vi "Mpemba_HotColdWarm.vi"(6 "RN":sgl, 8 "X0":sgl=0.5, 11 "Ring":i16(ring) items=["Cold", "Warm", "Hot"]) -> (3 "Xpot":sgl)   [LabVIEW 2019]
uses:
  <vilib>/Platform/TimedLoop/XDataNode/timing_clust.ctl
  <vilib>/Platform/TimedLoop/XDataNode/nitl_modes.ctl
  <vilib>/Platform/TimedLoop/XDataNode/wakeup.ctl
  <vilib>/rvi/Emulation/niFpgaGetClockAttributes.vi
  <vilib>/rvi/Emulation/niFpgaSctlEmulationGetInTimedLoop.vi
  <vilib>/rvi/Emulation/niFpgaEmulationReportErrorSimple.vi
  <vilib>/rvi/Emulation/niFpgaCriticalErrorInLSC.vi
  <vilib>/Platform/TimedLoop/XDataNode/XDataNode.xnode
  <vilib>/Platform/TimedLoop/XDataNode/XDNodeRunTimeDep.lvlib
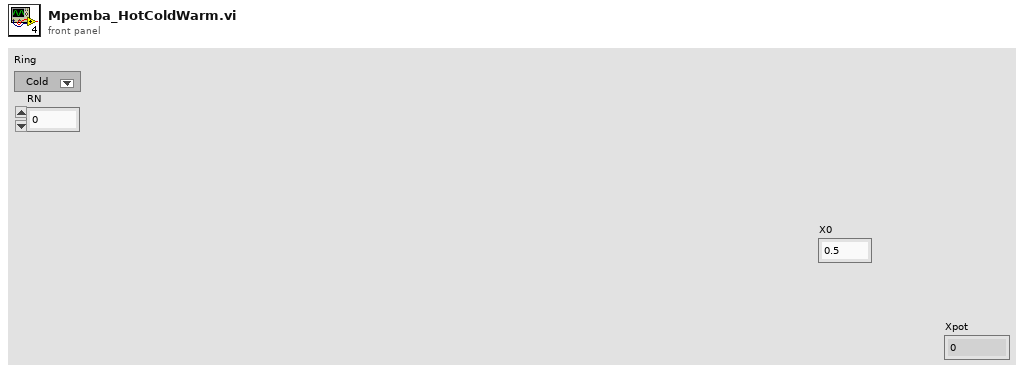
[diagram p1: front panel]
types:
  T1 = typedef "XDNodeRunTimeDep.lvlib/timing_clust.ctl" = cluster{"Expected End [f-1]":u64, "Actual End [f-1]":u64, "Finished Late? [f-1]":bool, "Expected End [i-1]":u64, "Actual End [i-1]":u64, "Finished Late? [i-1]":bool, "Expected Start [i]":u64, "Actual Start [i]":u64, "Expected Start [f]":u64, "Actual Start [f]":u64, "Source Name":string, "Structure Name":string, "Period":i64, "Deadline":i64, "Offset":i64, "Start":i64, "Priority":i32, "Timeout":i32, "Mode":T2, "Wakeup Reason":T3, "Error":errorcluster, "Source Type":string, "Secondary Source Type":string, "Global End Time":u64, "Global Start Time":u64, "Frame Duration":u64, "Iteration Duration":u64, "Assigned CPU":i32, "I/O Scan Engine Mode":u32}
  T2 = typedef "XDNodeRunTimeDep.lvlib/nitl_modes.ctl" = enum32{"No Change", "Process missed periods, maintain original phase", "Discard missed periods, maintain original phase", "Process missed periods, ignore original phase", "Discard missed periods, ignore original phase"}
  T3 = typedef "XDNodeRunTimeDep.lvlib/wakeup.ctl" = enum32{"Normal", "Aborted", "Asynchronous wakeup", "Timing source error", "Timed loop error", "Timeout"}
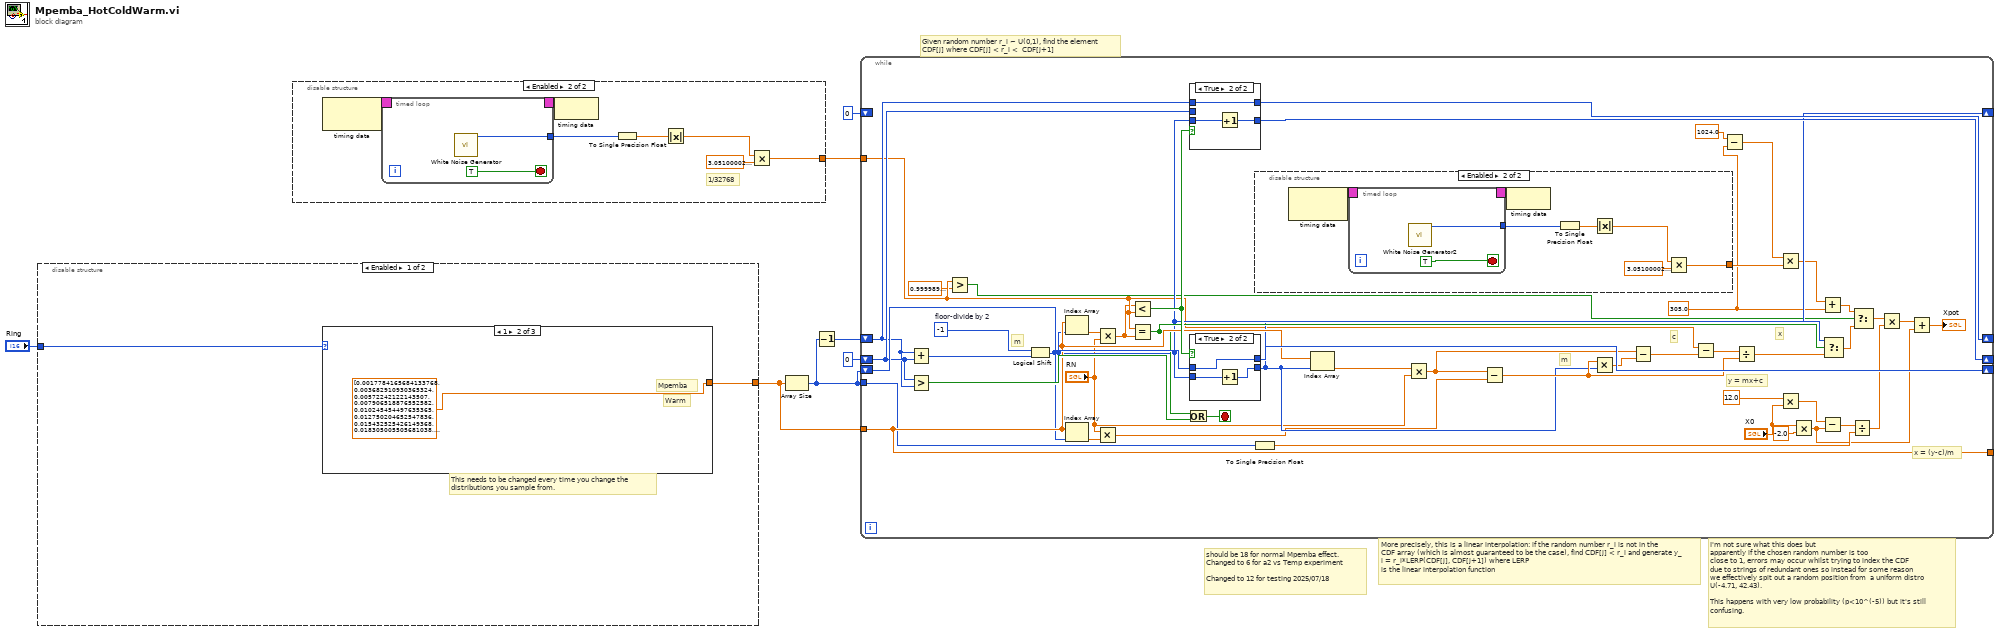
[diagram p0: block diagram]
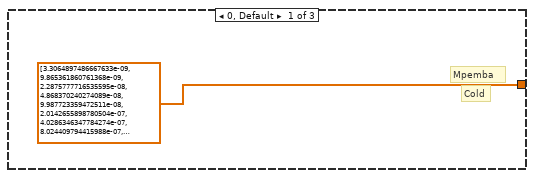
[diagram p2: hidden frame]
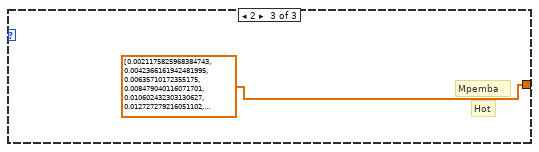
[diagram p3: hidden frame]
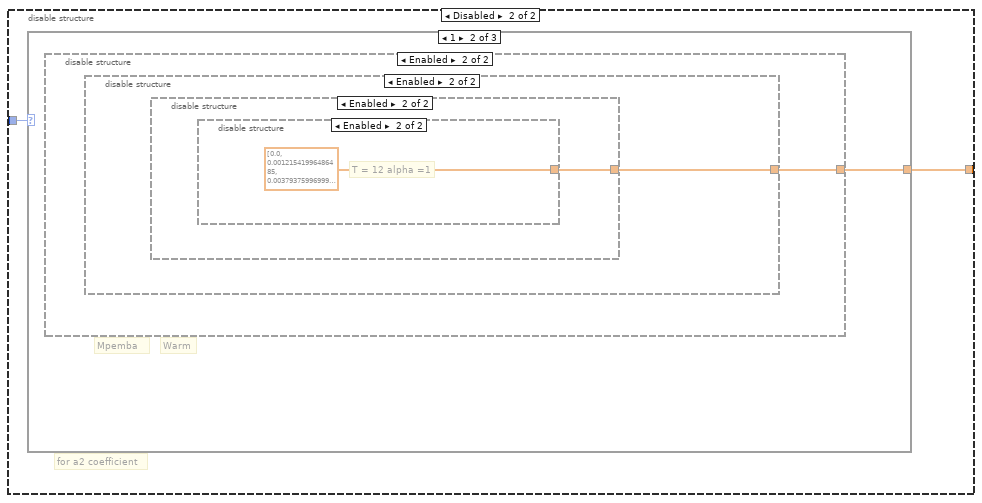
[diagram p4: hidden frame]
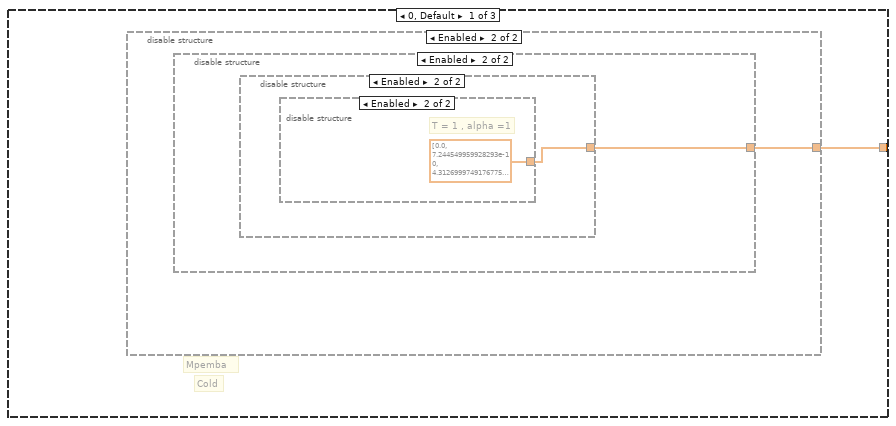
[diagram p5: hidden frame]
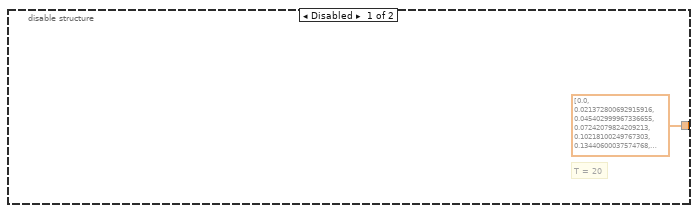
[diagram p6: hidden frame]
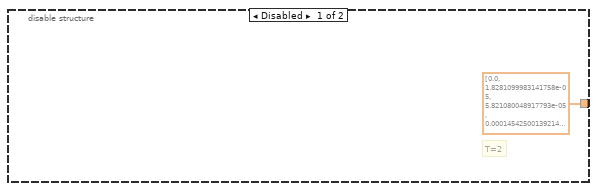
[diagram p7: hidden frame]
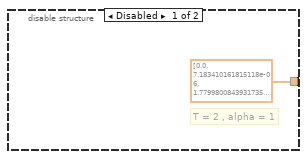
[diagram p8: hidden frame]
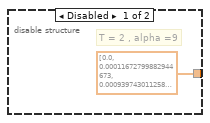
[diagram p9: hidden frame]
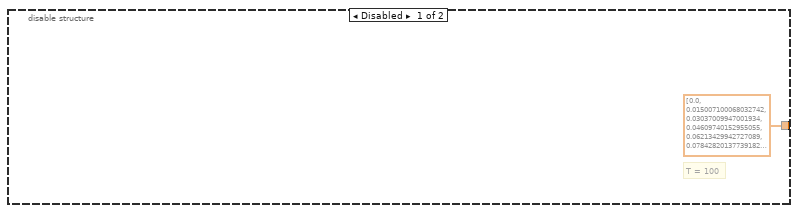
[diagram p10: hidden frame]
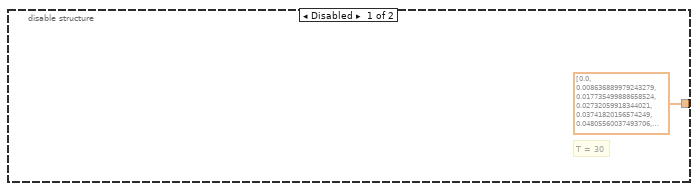
[diagram p11: hidden frame]
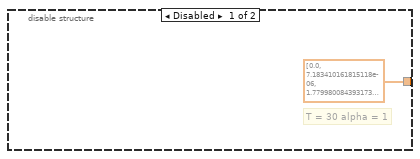
[diagram p12: hidden frame]
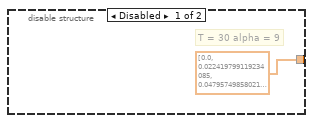
[diagram p13: hidden frame]
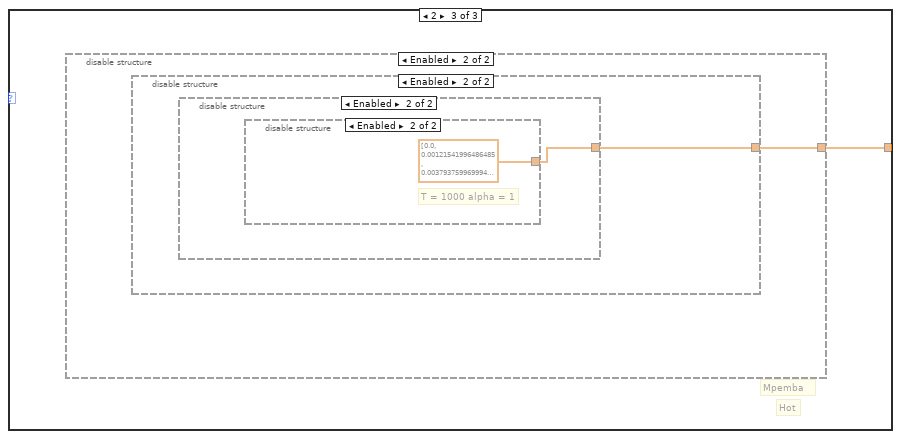
[diagram p14: hidden frame]
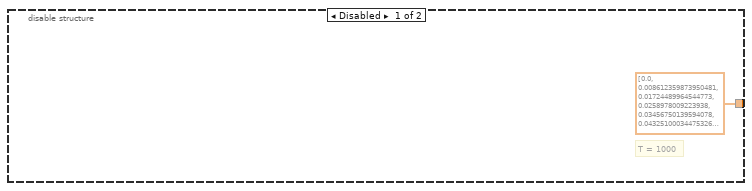
[diagram p15: hidden frame]
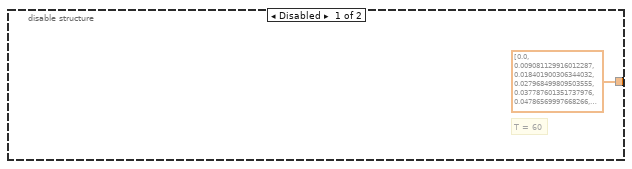
[diagram p16: hidden frame]
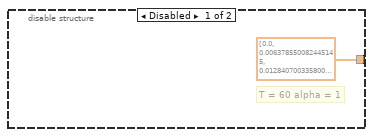
[diagram p17: hidden frame]
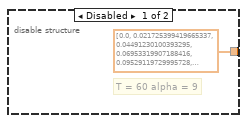
[diagram p18: hidden frame]
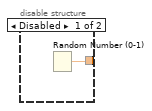
[diagram p19: hidden frame]
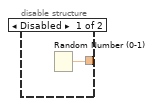
[diagram p20: hidden frame]
diagram:
  # "Given random number r_i ~ U(0,1), find the element\nCDF[j] where CDF[j] < r_i <  CDF[j+1]"
  # "I'm not sure what this does but\napparently if the chosen random number is too \nclose to 1, errors may occur whilst trying to index the CDF\ndue to strings of redundant ones so instead for some reason\nwe effectively spit out a random position from  a uniform distro\nU(-4.71, 42.43).\n\nThis happens with very low probability (p<10^(-5)) but it's still\nconfusing."
  # "More precisely, this is a linear interpolation: if the random number r_i is not in the\nCDF array (which is almost guaranteed to be the case), find CDF[j] < r_i and generate y_i = r_i*LERP(CDF[j], CDF[j+1]) where LERP\nis the linear interpolation function"
  # "should be 18 for normal Mpemba effect.\nChanged to 6 for a2 vs Temp experiment\n\nChanged to 12 for testing 2025/07/18"
  n1 = disable-structure shown="Enabled" {
    disable-tunnel: "Ring" -> [w9 w13]
    disable-tunnel: [w8 w14] -> w1
    frame Enabled {
      # "This needs to be changed every time you change the \ndistributions you sample from."
      n2 = case shown="1" w9 {
        tunnel: [sgl[] [3.3064897e-09, 9.865362e-09, 2.2875778e-08, 4.8683702e-08, 9.9877234e-08, 2.0142656e-07, 4.0286346e-07, 8.02441e-07, 1.5950573e-06, 3.1673194e-06, 6.286115e-06, 1.247267e-05, 2.4715764e-05, 4.8135003e-05, 9.1060996e-05, 0.00016657586, 0.0002942775, 0.00050219335, 0.0008286077, 0.0013234806, 0.0020490861, 0.0030795163, 0.004498784, 0.006397423, 0.008867702, 0.011997792, 0.015865415, 0.020531645, 0.026035521, 0.03239009, 0.039580304, 0.047562927, 0.0562685, 0.06560501, 0.075462855, 0.085720666, 0.0962513, 0.106927626, 0.11762765, 0.12823877, 0.13866088, 0.14880845, 0.15861152, 0.16801578, 0.17698202, 0.18548483, 0.19351119, 0.20105864, 0.20813352, 0.2147492, 0.22092445, 0.22668195, 0.23204707, 0.23704672, 0.24170859, 0.24606037, 0.25012928, 0.25394168, 0.25752282, 0.2608967, 0.26408604, 0.2671121, 0.2699949, 0.27275333, 0.27540496, 0.2779665, 0.28045377, 0.28288183, 0.28526524, 0.28761804, 0.2899542, 0.2922874, 0.29463166, 0.2970011, 0.29941046, 0.3018751, 0.30441135, 0.30703667, 0.30977, 0.31263185, 0.31564495, 0.31883422, 0.32222733, 0.3258551, 0.32975185, 0.33395582, 0.33850968, 0.34346086, 0.34886217, 0.354772, 0.36125463, 0.36838052, 0.37622622, 0.3848741, 0.3944119, 0.40493152, 0.4165278, 0.42929626, 0.44333023, 0.4587175, 0.4755356, 0.49384695, 0.5136926, 0.535086, 0.558006, 0.5823905, 0.60813034, 0.63506484, 0.6629795, 0.69160587, 0.72062594, 0.7496793, 0.77837545, 0.8063088, 0.83307797, 0.85830593, 0.8816607, 0.9028746, 0.92175883, 0.93821377, 0.95223135, 0.9638909, 0.9733483, 0.9808191, 0.9865588, 0.9908417, 0.9939414, 0.99611413, 0.9975871, 0.99855137, 0.9991601, 0.99953, 0.9997462, 0.9998674, 0.99993247, 0.99996597, 0.99998283, 0.99999136, 0.99999565, 0.9999978, 0.99999887, 0.99999946, 0.9999997, 0.9999999, 0.99999994, 0.99999994, 1.0, 1.0, 1.0, 1.0, 1.0, 1.0, 1.0, 1.0, 1.0, 1.0, 1.0, 1.0, 1.0, 1.0, 1.0, 1.0, 1.0, 1.0, 1.0, 1.0, 1.0, 1.0, 1.0, 1.0, 1.0, 1.0, 1.0, 1.0, 1.0, 1.0, 1.0, 1.0, 1.0, 1.0, 1.0, 1.0, 1.0, 1.0, 1.0, 1.0, 1.0, 1.0, 1.0, 1.0, 1.0, 1.0, 1.0, 1.0, 1.0, 1.0, 1.0, 1.0, 1.0, 1.0, 1.0, 1.0, 1.0, 1.0, 1.0, 1.0, 1.0, 1.0, 1.0, 1.0, 1.0, 1.0, 1.0, 1.0, 1.0, 1.0, 1.0, 1.0, 1.0, 1.0, 1.0, 1.0, 1.0, 1.0, 1.0, 1.0, 1.0, 1.0, 1.0, 1.0, 1.0, 1.0, 1.0, 1.0, 1.0, 1.0, 1.0, 1.0, 1.0, 1.0, 1.0, 1.0, 1.0, 1.0, 1.0, 1.0, 1.0, 1.0, 1.0, 1.0, 1.0, 1.0, 1.0, 1.0, 1.0, 1.0, 1.0, 1.0, 1.0, 1.0, 1.0, 1.0, 1.0, 1.0, 1.0, 1.0, 1.0, 1.0, 1.0, 1.0, 1.0, 1.0, 1.0, 1.0, 1.0, 1.0, 1.0, 1.0, 1.0, 1.0, 1.0, 1.0, 1.0, 1.0, 1.0, 1.0, 1.0, 1.0, 1.0, 1.0, 1.0, 1.0, 1.0, 1.0, 1.0, 1.0, 1.0, 1.0, 1.0, 1.0, 1.0, 1.0, 1.0, 1.0, 1.0, 1.0, 1.0, 1.0, 1.0, 1.0, 1.0, 1.0, 1.0, 1.0, 1.0, 1.0, 1.0, 1.0, 1.0, 1.0, 1.0, 1.0, 1.0, 1.0, 1.0, 1.0, 1.0, 1.0, 1.0, 1.0, 1.0, 1.0, 1.0, 1.0, 1.0, 1.0, 1.0, 1.0, 1.0, 1.0, 1.0, 1.0, 1.0, 1.0, 1.0, 1.0, 1.0, 1.0, 1.0, 1.0, 1.0, 1.0, 1.0, 1.0, 1.0, 1.0, 1.0, 1.0, 1.0, 1.0, 1.0, 1.0, 1.0, 1.0, 1.0, 1.0, 1.0, 1.0, 1.0, 1.0, 1.0, 1.0, 1.0, 1.0, 1.0, 1.0, 1.0, 1.0, 1.0, 1.0, 1.0, 1.0, 1.0, 1.0, 1.0, 1.0, 1.0, 1.0, 1.0, 1.0, 1.0, 1.0, 1.0, 1.0, 1.0, 1.0, 1.0, 1.0, 1.0, 1.0, 1.0, 1.0, 1.0, 1.0, 1.0, 1.0, 1.0, 1.0, 1.0, 1.0, 1.0, 1.0, 1.0, 1.0, 1.0, 1.0, 1.0, 1.0, 1.0, 1.0, 1.0, 1.0, 1.0, 1.0, 1.0, 1.0, 1.0, 1.0, 1.0, 1.0, 1.0, 1.0, 1.0, 1.0, 1.0, 1.0, 1.0, 1.0, 1.0, 1.0, 1.0, 1.0, 1.0, 1.0, 1.0, 1.0, 1.0, 1.0, 1.0, 1.0, 1.0, 1.0, 1.0, 1.0, 1.0, 1.0, 1.0, 1.0, 1.0, 1.0, 1.0, 1.0, 1.0, 1.0, 1.0, 1.0, 1.0, 1.0, 1.0, 1.0, 1.0, 1.0, 1.0, 1.0, 1.0, 1.0, 1.0, 1.0, 1.0, 1.0, 1.0, 1.0, 1.0, 1.0, 1.0, 1.0, 1.0, 1.0, 1.0, 1.0, 1.0, 1.0, 1.0, 1.0, 1.0, 1.0, 1.0, 1.0, 1.0, 1.0, 1.0, 1.0, 1.0, 1.0, 1.0, 1.0, 1.0, 1.0, 1.0, 1.0, 1.0, 1.0, 0.0, 0.0] ("Array") sgl[] [0.0017784166, 0.003682911, 0.005722421, 0.007906519, 0.0102454545, 0.012750205, 0.015432525, 0.018305006, 0.021381123, 0.024675317, 0.02820305, 0.031980872, 0.03602557, 0.040341295, 0.044926606, 0.049778376, 0.054891855, 0.060260758, 0.065877356, 0.07173262, 0.07781631, 0.084117144, 0.090622984, 0.09732092, 0.10419748, 0.11123878, 0.11843064, 0.12575877, 0.1332089, 0.14076687, 0.1484188, 0.15615115, 0.16395082, 0.17180526, 0.17970249, 0.1876312, 0.19558074, 0.20354122, 0.21150346, 0.21945906, 0.22740036, 0.23532051, 0.24321334, 0.25107348, 0.2588962, 0.2666775, 0.27441406, 0.2821032, 0.28974277, 0.29733124, 0.3048676, 0.31235138, 0.3197825, 0.32716137, 0.33448884, 0.34176603, 0.34899446, 0.356176, 0.3633127, 0.37040702, 0.37746152, 0.38447905, 0.39146265, 0.39841548, 0.40534094, 0.4122425, 0.41912377, 0.4259885, 0.43284047, 0.43968362, 0.44652188, 0.4533593, 0.46019995, 0.46704793, 0.47390732, 0.48078233, 0.48767704, 0.4945956, 0.5015421, 0.5085206, 0.5155351, 0.52258956, 0.52968794, 0.5368339, 0.54403114, 0.55128324, 0.5585935, 0.56596524, 0.57340133, 0.58090466, 0.58847773, 0.5961228, 0.6038418, 0.6116363, 0.6195075, 0.6274562, 0.6354827, 0.64358693, 0.6517681, 0.66002494, 0.6683555, 0.6767572, 0.68522686, 0.6937603, 0.70235276, 0.7109986, 0.7196914, 0.72842366, 0.7371872, 0.7459729, 0.7547705, 0.7635692, 0.7723569, 0.7811211, 0.78984797, 0.7985233, 0.80713195, 0.81565815, 0.82408583, 0.83239824, 0.84057844, 0.8486093, 0.8564739, 0.8641552, 0.8716366, 0.8789022, 0.8859366, 0.8927255, 0.8992556, 0.9055147, 0.91149247, 0.9171798, 0.92256963, 0.9276564, 0.9324368, 0.9369095, 0.9410861, 0.9449862, 0.9486281, 0.952029, 0.95520467, 0.9581701, 0.9609393, 0.9635251, 0.96593976, 0.96819454, 0.9703001, 0.9722662, 0.9741022, 0.9758166, 0.9774176, 0.97891253, 0.98030853, 0.9816121, 0.9828294, 0.98396605, 0.98502755, 0.9860187, 0.98694426, 0.9878086, 0.98861563, 0.9893693, 0.990073, 0.9907302, 0.99134386, 0.9919169, 0.992452, 0.9929517, 0.9934183, 0.993854, 0.99426085, 0.99464077, 0.9949956, 0.9953269, 0.9956362, 0.9959251, 0.99619484, 0.9964468, 0.996682, 0.99690163, 0.99710673, 0.9972983, 0.9974771, 0.9976442, 0.9978001, 0.9979457, 0.99808174, 0.9982087, 0.9983273, 0.99843806, 0.9985415, 0.998638, 0.99872816, 0.9988124, 0.998891, 0.9989644, 0.999033, 0.999097, 0.9991568, 0.99921256, 0.9992647, 0.99931335, 0.99935883, 0.9994013, 0.9994409, 0.9994779, 0.9995125, 0.99954474, 0.9995749, 0.99960303, 0.9996293, 0.9996539, 0.99967676, 0.99969816, 0.9997181, 0.9997368, 0.99975425, 0.9997705, 0.9997857, 0.9997999, 0.99981314, 0.9998255, 0.99983704, 0.9998478, 0.9998579, 0.9998673, 0.9998761, 0.9998843, 0.99989194, 0.9998991, 0.99990577, 0.999912, 0.99991786, 0.9999233, 0.99992836, 0.9999331, 0.99993753, 0.99994165, 0.9999455, 0.99994916, 0.9999525, 0.99995565, 0.9999586, 0.9999613, 0.9999639, 0.99996626, 0.9999685, 0.9999706, 0.9999725, 0.99997437, 0.99997604, 0.99997765, 0.99997914, 0.9999805, 0.9999818, 0.999983, 0.99998415, 0.99998516, 0.9999862, 0.99998707, 0.99998796, 0.99998873, 0.99998945, 0.99999017, 0.9999908, 0.9999914, 0.999992, 0.99999255, 0.999993, 0.9999935, 0.9999939, 0.99999434, 0.9999947, 0.99999505, 0.99999535, 0.9999957, 0.99999595, 0.99999624, 0.9999965, 0.9999967, 0.99999696, 0.99999714, 0.9999973, 0.9999975, 0.9999977, 0.9999978, 0.999998, 0.9999981, 0.9999982, 0.99999833, 0.99999845, 0.99999857, 0.9999986, 0.99999875, 0.9999988, 0.9999989, 0.999999, 0.99999905, 0.9999991, 0.99999917, 0.9999992, 0.9999993, 0.99999934, 0.99999934, 0.9999994, 0.99999946, 0.99999946, 0.9999995, 0.9999995, 0.9999996, 0.9999996, 0.99999964, 0.99999964, 0.9999997, 0.9999997, 0.9999997, 0.99999976, 0.99999976, 0.99999976, 0.99999976, 0.9999998, 0.9999998, 0.9999998, 0.9999998, 0.9999998, 0.9999999, 0.9999999, 0.9999999, 0.9999999, 0.9999999, 0.9999999, 0.9999999, 0.99999994, 0.99999994, 0.99999994, 0.99999994, 0.99999994, 0.99999994, 0.99999994, 0.99999994, 0.99999994, 0.99999994, 0.99999994, 0.99999994, 0.99999994, 0.99999994, 0.99999994, 0.99999994, 1.0, 1.0, 1.0, 1.0, 1.0, 1.0, 1.0, 1.0, 1.0, 1.0, 1.0, 1.0, 1.0, 1.0, 1.0, 1.0, 1.0, 1.0, 1.0, 1.0, 1.0, 1.0, 1.0, 1.0, 1.0, 1.0, 1.0, 1.0, 1.0, 1.0, 1.0, 1.0, 1.0, 1.0, 1.0, 1.0, 1.0, 1.0, 1.0, 1.0, 1.0, 1.0, 1.0, 1.0, 1.0, 1.0, 1.0, 1.0, 1.0, 1.0, 1.0, 1.0, 1.0, 1.0, 1.0, 1.0, 1.0, 1.0, 1.0, 1.0, 1.0, 1.0, 1.0, 1.0, 1.0, 1.0, 1.0, 1.0, 1.0, 1.0, 1.0, 1.0, 1.0, 1.0, 1.0, 1.0, 1.0, 1.0, 1.0, 1.0, 1.0, 1.0, 1.0, 1.0, 1.0, 1.0, 1.0, 1.0, 1.0, 1.0, 1.0, 1.0, 1.0, 1.0, 1.0, 1.0, 1.0, 1.0, 1.0, 1.0, 1.0, 1.0, 1.0, 1.0, 1.0, 1.0, 1.0, 1.0, 1.0, 1.0, 1.0, 1.0, 1.0, 1.0, 1.0, 1.0, 1.0, 1.0, 1.0, 1.0, 1.0, 1.0, 1.0, 1.0, 1.0, 1.0, 1.0, 1.0, 1.0, 1.0, 1.0, 1.0, 1.0, 1.0, 1.0, 1.0, 1.0, 1.0, 1.0, 1.0, 1.0, 1.0, 1.0, 1.0, 1.0, 1.0, 1.0, 1.0, 1.0, 1.0, 1.0, 1.0, 1.0, 1.0, 1.0, 1.0, 1.0, 1.0, 1.0, 1.0, 1.0, 1.0, 1.0, 1.0, 0.0, 0.0] ("Array") sgl[] [0.0021175826, 0.004236616, 0.0063571017, 0.00847904, 0.010602432, 0.012727279, 0.014853583, 0.016981343, 0.01911056, 0.021241236, 0.023373373, 0.02550697, 0.027642025, 0.029778464, 0.031916197, 0.03405514, 0.036195207, 0.038336314, 0.040478393, 0.04262136, 0.044765145, 0.046909686, 0.049054913, 0.051200762, 0.053347178, 0.0554941, 0.05764148, 0.05978926, 0.061937395, 0.06408584, 0.06623455, 0.068383485, 0.070532605, 0.072681874, 0.07483126, 0.07698074, 0.07913027, 0.08127982, 0.08342939, 0.08557893, 0.08772844, 0.089877896, 0.09202727, 0.09417655, 0.09632574, 0.09847481, 0.10062376, 0.10277257, 0.104921244, 0.107069775, 0.10921816, 0.11136639, 0.11351447, 0.1156624, 0.11781018, 0.11995781, 0.1221053, 0.12425265, 0.12639986, 0.12854694, 0.1306939, 0.13284075, 0.1349875, 0.13713415, 0.13928072, 0.14142722, 0.14357364, 0.14572002, 0.14786637, 0.15001267, 0.15215896, 0.15430526, 0.15645157, 0.15859789, 0.16074425, 0.16289066, 0.16503714, 0.16718368, 0.16933031, 0.17147705, 0.17362389, 0.17577085, 0.17791794, 0.18006518, 0.18221258, 0.18436013, 0.18650787, 0.18865578, 0.19080387, 0.19295216, 0.19510065, 0.19724934, 0.19939823, 0.20154734, 0.20369665, 0.20584618, 0.20799592, 0.21014586, 0.21229601, 0.21444635, 0.21659689, 0.21874762, 0.22089851, 0.22304955, 0.22520076, 0.2273521, 0.22950354, 0.23165509, 0.23380673, 0.2359584, 0.23811011, 0.24026182, 0.2424135, 0.24456514, 0.24671668, 0.24886808, 0.25101933, 0.25317037, 0.25532115, 0.25747165, 0.25962177, 0.26177153, 0.2639208, 0.26606962, 0.26821783, 0.27036545, 0.27251235, 0.27465847, 0.2768038, 0.2789482, 0.2810916, 0.28323394, 0.28537515, 0.2875151, 0.28965372, 0.2917909, 0.29392666, 0.29606092, 0.29819375, 0.3003251, 0.302455, 0.30458343, 0.30671042, 0.30883595, 0.31096002, 0.31308264, 0.3152038, 0.3173235, 0.31944177, 0.32155856, 0.3236739, 0.32578784, 0.3279003, 0.3300113, 0.33212087, 0.334229, 0.3363357, 0.33844092, 0.34054473, 0.34264708, 0.344748, 0.34684747, 0.34894553, 0.35104212, 0.35313728, 0.35523102, 0.35732335, 0.3594142, 0.36150363, 0.36359164, 0.36567822, 0.36776337, 0.3698471, 0.37192938, 0.37401026, 0.3760897, 0.37816772, 0.3802443, 0.3823195, 0.38439324, 0.38646558, 0.3885365, 0.39060602, 0.3926741, 0.39474076, 0.396806, 0.39886984, 0.40093225, 0.40299326, 0.40505287, 0.40711105, 0.40916783, 0.4112232, 0.41327718, 0.41532972, 0.41738087, 0.41943064, 0.421479, 0.42352593, 0.42557147, 0.4276156, 0.42965835, 0.4316997, 0.43373963, 0.43577817, 0.43781534, 0.43985108, 0.44188544, 0.4439184, 0.44595, 0.4479802, 0.450009, 0.45203638, 0.4540624, 0.45608705, 0.45811027, 0.46013215, 0.46215263, 0.4641717, 0.4661894, 0.46820575, 0.4702207, 0.47223428, 0.47424647, 0.47625726, 0.47826672, 0.48027477, 0.48228145, 0.4842868, 0.48629072, 0.48829326, 0.49029446, 0.49229428, 0.49429274, 0.49628985, 0.49828556, 0.5002799, 0.5022729, 0.50426453, 0.5062548, 0.5082437, 0.5102312, 0.5122174, 0.5142022, 0.51618564, 0.51816773, 0.5201485, 0.52212787, 0.5241059, 0.5260826, 0.5280579, 0.53003186, 0.5320045, 0.5339757, 0.53594565, 0.5379142, 0.53988147, 0.54184735, 0.54381186, 0.54577506, 0.5477369, 0.54969734, 0.55165654, 0.5536143, 0.5555708, 0.55752593, 0.5594797, 0.5614322, 0.5633833, 0.56533307, 0.56728154, 0.56922865, 0.5711744, 0.57311887, 0.575062, 0.5770038, 0.5789442, 0.5808833, 0.58282113, 0.5847576, 0.58669275, 0.58862656, 0.59055907, 0.59249026, 0.5944201, 0.59634864, 0.59827584, 0.6002017, 0.6021263, 0.60404956, 0.60597146, 0.6078921, 0.6098114, 0.6117294, 0.6136461, 0.6155614, 0.6174755, 0.6193882, 0.6212997, 0.62320983, 0.6251186, 0.62702614, 0.62893236, 0.63083726, 0.63274086, 0.63464314, 0.6365441, 0.6384438, 0.6403422, 0.6422393, 0.64413506, 0.64602953, 0.64792275, 0.64981467, 0.65170527, 0.65359455, 0.6554826, 0.6573693, 0.6592547, 0.66113883, 0.6630217, 0.6649033, 0.6667835, 0.66866255, 0.6705402, 0.6724166, 0.67429173, 0.6761656, 0.6780382, 0.6799094, 0.68177944, 0.68364817, 0.6855156, 0.68738174, 0.6892466, 0.6911102, 0.69297254, 0.6948336, 0.69669336, 0.6985519, 0.7004091, 0.7022651, 0.70411974, 0.7059732, 0.7078253, 0.7096762, 0.7115258, 0.7133742, 0.7152213, 0.71706706, 0.71891165, 0.7207549, 0.72259694, 0.7244377, 0.72627723, 0.7281155, 0.72995245, 0.7317882, 0.73362267, 0.7354559, 0.7372879, 0.7391186, 0.740948, 0.7427762, 0.74460316, 0.74642885, 0.74825335, 0.75007653, 0.75189847, 0.75371915, 0.75553864, 0.7573568, 0.7591738, 0.76098955, 0.76280403, 0.76461726, 0.76642925, 0.76824003, 0.7700495, 0.7718578, 0.77366483, 0.7754707, 0.7772752, 0.77907854, 0.78088063, 0.7826815, 0.7844811, 0.7862795, 0.7880767, 0.78987265, 0.79166734, 0.7934608, 0.79525304, 0.79704404, 0.79883385, 0.8006224, 0.80240977, 0.8041959, 0.8059808, 0.8077645, 0.80954695, 0.8113282, 0.81310815, 0.814887, 0.8166645, 0.8184409, 0.82021606, 0.82198995, 0.8237627, 0.82553416, 0.8273045, 0.82907355, 0.8308414, 0.83260804, 0.83437353, 0.8361378, 0.83790076, 0.8396626, 0.8414232, 0.8431826, 0.84494084, 0.8466978, 0.8484536, 0.8502082, 0.8519616, 0.8537138, 0.85546476, 0.85721457, 0.8589632, 0.86071056, 0.8624568, 0.8642018, 0.8659456, 0.8676882, 0.86942965, 0.87116987, 0.8729089, 0.8746468, 0.8763834, 0.8781189, 0.8798532, 0.88158625, 0.8833182, 0.88504887, 0.8867784, 0.88850677, 0.89023393, 0.89195997, 0.89368474, 0.8954084, 0.8971308, 0.89885205, 0.9005722, 0.90229106, 0.9040088, 0.90572536, 0.9074407, 0.90915495, 0.910868, 0.91257983, 0.91429055, 0.91600007, 0.9177084, 0.9194156, 0.9211216, 0.9228264, 0.9245301, 0.9262326, 0.92793393, 0.9296341, 0.9313331, 0.93303096, 0.93472767, 0.9364232, 0.9381175, 0.93981075, 0.94150275, 0.9431937, 0.9448834, 0.94657195, 0.94825935, 0.9499456, 0.9516307, 0.95331466, 0.9549975, 0.9566791, 0.9583596, 0.96003896, 0.9617171, 0.96339417, 0.96507007, 0.96674484, 0.9684184, 0.97009087, 0.9717622, 0.97343236, 0.97510135, 0.97676927, 0.978436, 0.9801016, 0.98176605, 0.9834294, 0.9850915, 0.98675257, 0.9884125, 0.99007124, 0.99172884, 0.9933854, 0.9950407, 0.9966949, 0.99834806, 1.0, 0.0, 0.0] ("Array")] -> w8
        frame 0, Default {
          # "Mpemba"
          # "Cold"
        }
        frame 1 {
          # "Mpemba"
          # "Warm"
        }
        frame 2 {
          # "Mpemba"
          # "Hot"
        }
      }
    }
    frame Disabled {
      # "for a2 coefficient"
      n3 = case shown="1" w13 {
        tunnel: [w15 w24 w33] -> w14
        frame 0, Default {
          # "Mpemba"
          # "Cold"
          n4 = disable-structure shown="Enabled" {
            disable-tunnel: [sgl[] [0.0, 0.0213728, 0.045403, 0.0724208, 0.102181, 0.134406, 0.168527, 0.203294, 0.237827, 0.271636, 0.304566, 0.336711, 0.368335, 0.399797, 0.431501, 0.46385, 0.49719, 0.531749, 0.567555, 0.604331, 0.641406, 0.677659, 0.712252, 0.744072, 0.772373, 0.797545, 0.819933, 0.839845, 0.857555, 0.873307, 0.887317, 0.899778, 0.910861, 0.920718, 0.929485, 0.937283, 0.944219, 0.950387, 0.955874, 0.960753, 0.965093, 0.968954, 0.972387, 0.975441, 0.978156, 0.980572, 0.982721, 0.984632, 0.986331, 0.987843, 0.989187, 0.990383, 0.991447, 0.992393, 0.993234, 0.993982, 0.994648, 0.99524, 0.995766, 0.996235, 0.996651, 0.997022, 0.997351, 0.997644, 0.997905, 0.998137, 0.998343, 0.998526, 0.998689, 0.998834, 0.998964, 0.999078, 0.99918, 0.999271, 0.999352, 0.999424, 0.999488, 0.999544, 0.999595, 0.99964, 0.99968, 0.999715, 0.999747, 0.999775, 0.9998, 0.999822, 0.999842, 0.99986, 0.999875, 0.999889, 0.999902, 0.999913, 0.999923, 0.999931, 0.999939, 0.999946, 0.999952, 0.999957, 0.999962, 0.999967, 0.99997, 0.999974, 0.999977, 0.99998, 0.999982, 0.999984, 0.999986, 0.999988, 0.999989, 0.999991, 0.999992, 0.999993, 0.999994, 0.999995, 0.999995, 0.999996, 0.999997, 0.999997, 0.999998, 0.999998, 0.999998, 0.999999, 0.999999, 0.999999, 0.999999, 1.0, 1.0, 1.0] ("Init Data Out") w17] -> w15
            frame Disabled {
              # "T = 20"
            }
            frame Enabled {
              n5 = disable-structure shown="Enabled" {
                disable-tunnel: [sgl[] [0.0, 1.82811e-05, 5.82108e-05, 0.000145425, 0.000335919, 0.000751995, 0.00163728, 0.00336872, 0.00643385, 0.0113875, 0.0187564, 0.0289264, 0.0420484, 0.0579922, 0.0763639, 0.0965741, 0.117935, 0.139759, 0.161435, 0.182478, 0.202546, 0.221436, 0.239063, 0.255433, 0.270621, 0.284744, 0.297945, 0.310381, 0.322214, 0.333607, 0.344725, 0.355731, 0.366794, 0.378089, 0.389801, 0.402131, 0.415301, 0.429557, 0.445172, 0.462448, 0.481709, 0.503297, 0.527545, 0.554752, 0.585135, 0.61877, 0.655517, 0.694956, 0.736325, 0.778508, 0.820083, 0.85945, 0.895035, 0.925537, 0.950157, 0.968733, 0.981736, 0.990113, 0.99504, 0.997663, 0.99893, 0.99951, 0.999776, 0.999897, 0.999953, 0.999978, 0.99999, 0.999995, 0.999998, 0.999999, 1.0, 1.0, 1.0, 1.0, 1.0, 1.0, 1.0, 1.0, 1.0, 1.0, 1.0, 1.0, 1.0, 1.0, 1.0, 1.0, 1.0, 1.0, 1.0, 1.0, 1.0, 1.0, 1.0, 1.0, 1.0, 1.0, 1.0, 1.0, 1.0, 1.0, 1.0, 1.0, 1.0, 1.0, 1.0, 1.0, 1.0, 1.0, 1.0, 1.0, 1.0, 1.0, 1.0, 1.0, 1.0, 1.0, 1.0, 1.0, 1.0, 1.0, 1.0, 1.0, 1.0, 1.0, 1.0, 1.0, 1.0, 1.0] ("Init Data Out") w19] -> w17
                frame Disabled {
                  # "T=2"
                }
                frame Enabled {
                  n6 = disable-structure shown="Enabled" {
                    disable-tunnel: [sgl[] [0.0, 7.18341e-06, 1.77998e-05, 3.34898e-05, 5.66781e-05, 9.09483e-05, 0.000141596, 0.000216449, 0.000327074, 0.000490568, 0.000732196, 0.00108818, 0.00160286, 0.00232691, 0.00331916, 0.00464534, 0.00637594, 0.00858334, 0.0113384, 0.0147065, 0.018744, 0.0234947, 0.0289869, 0.0352312, 0.0422199, 0.0499271, 0.0583093, 0.0673079, 0.0768517, 0.0868599, 0.0972457, 0.107919, 0.118792, 0.129776, 0.140791, 0.151763, 0.162627, 0.173325, 0.18381, 0.194044, 0.203998, 0.21365, 0.222987, 0.232003, 0.240696, 0.24907, 0.257133, 0.264897, 0.272375, 0.279584, 0.286542, 0.293267, 0.299778, 0.306097, 0.312243, 0.318237, 0.324099, 0.32985, 0.33551, 0.341101, 0.346642, 0.352154, 0.357659, 0.363176, 0.368728, 0.374337, 0.380026, 0.385817, 0.391736, 0.397808, 0.40406, 0.41052, 0.417219, 0.424187, 0.431457, 0.439066, 0.447049, 0.455444, 0.464293, 0.473636, 0.483515, 0.493973, 0.505054, 0.516798, 0.529244, 0.54243, 0.556386, 0.571137, 0.586698, 0.603073, 0.620255, 0.63822, 0.656925, 0.676309, 0.696287, 0.716756, 0.737584, 0.758622, 0.779699, 0.800628, 0.821208, 0.841235, 0.860504, 0.878821, 0.896007, 0.911909, 0.926408, 0.939421, 0.950908, 0.960869, 0.969349, 0.976426, 0.982213, 0.986842, 0.990462, 0.993225, 0.995283, 0.996775, 0.997829, 0.998552, 0.999042, 0.999373, 0.999597, 0.999749, 0.999852, 0.999921, 0.999968, 1.0] ("Init Data Out") w21] -> w19
                    frame Disabled {
                      # "T = 2 , alpha = 1"
                    }
                    frame Enabled {
                      n7 = disable-structure shown="Enabled" {
                        disable-tunnel: [sgl[] [0.0, 0.000116728, 0.000939743, 0.00543746, 0.0201801, 0.0512956, 0.0978339, 0.151563, 0.20343, 0.248501, 0.286144, 0.318051, 0.34667, 0.374589, 0.404577, 0.439926, 0.4848, 0.544122, 0.622008, 0.717698, 0.820325, 0.909305, 0.966774, 0.992101, 0.99888, 0.999841, 0.999977, 0.999997, 1.0, 1.0, 1.0, 1.0, 1.0, 1.0, 1.0, 1.0, 1.0, 1.0, 1.0, 1.0, 1.0, 1.0, 1.0, 1.0, 1.0, 1.0, 1.0, 1.0, 1.0, 1.0, 1.0, 1.0, 1.0, 1.0, 1.0, 1.0, 1.0, 1.0, 1.0, 1.0, 1.0, 1.0, 1.0, 1.0, 1.0, 1.0, 1.0, 1.0, 1.0, 1.0, 1.0, 1.0, 1.0, 1.0, 1.0, 1.0, 1.0, 1.0, 1.0, 1.0, 1.0, 1.0, 1.0, 1.0, 1.0, 1.0, 1.0, 1.0, 1.0, 1.0, 1.0, 1.0, 1.0, 1.0, 1.0, 1.0, 1.0, 1.0, 1.0, 1.0, 1.0, 1.0, 1.0, 1.0, 1.0, 1.0, 1.0, 1.0, 1.0, 1.0, 1.0, 1.0, 1.0, 1.0, 1.0, 1.0, 1.0, 1.0, 1.0, 1.0, 1.0, 1.0, 1.0, 1.0, 1.0, 1.0, 1.0, 1.0] ("Init Data Out") sgl[] [0.0, 7.24455e-10, 4.3127e-09, 1.7625e-08, 6.33566e-08, 2.09223e-07, 6.42359e-07, 1.84285e-06, 4.95654e-06, 1.2533e-05, 2.98716e-05, 6.72795e-05, 0.00014355, 0.000290853, 0.000560954, 0.00103223, 0.00181642, 0.00306355, 0.00496314, 0.00774017, 0.0116446, 0.0169346, 0.0238551, 0.0326133, 0.0433563, 0.0561516, 0.0709756, 0.0877112, 0.106153, 0.126023, 0.146989, 0.168687, 0.190746, 0.212812, 0.234557, 0.2557, 0.276012, 0.295314, 0.313485, 0.33045, 0.346176, 0.360668, 0.373958, 0.386099, 0.39716, 0.407218, 0.416356, 0.424657, 0.432205, 0.439077, 0.44535, 0.451091, 0.456366, 0.461233, 0.465744, 0.469948, 0.473889, 0.477605, 0.481132, 0.484503, 0.487749, 0.490895, 0.49397, 0.496997, 0.5, 0.503003, 0.50603, 0.509105, 0.512252, 0.515497, 0.518868, 0.522396, 0.526112, 0.530052, 0.534256, 0.538768, 0.543634, 0.548909, 0.554651, 0.560923, 0.567795, 0.575343, 0.583644, 0.592782, 0.60284, 0.613901, 0.626042, 0.639332, 0.653824, 0.669551, 0.686515, 0.704686, 0.723989, 0.7443, 0.765443, 0.787189, 0.809254, 0.831314, 0.853012, 0.873977, 0.893847, 0.912289, 0.929025, 0.943849, 0.956644, 0.967387, 0.976145, 0.983066, 0.988356, 0.99226, 0.995037, 0.996937, 0.998184, 0.998968, 0.999439, 0.999709, 0.999857, 0.999933, 0.99997, 0.999988, 0.999995, 0.999998, 1.0, 1.0, 1.0, 1.0, 1.0, 1.0] ("Init Data Out")] -> w21
                        frame Disabled {
                          # "T = 2 , alpha =9"
                        }
                        frame Enabled {
                          # "T = 1 , alpha =1"
                        }
                      }
                    }
                  }
                }
              }
            }
          }
        }
        frame 1 {
          # "Mpemba"
          # "Warm"
          n8 = disable-structure shown="Enabled" {
            disable-tunnel: [sgl[] [0.0, 0.0150071, 0.0303701, 0.0460974, 0.0621343, 0.0784282, 0.0949112, 0.111457, 0.12798, 0.144433, 0.160799, 0.177087, 0.193322, 0.20954, 0.225783, 0.242091, 0.258498, 0.275023, 0.291666, 0.308398, 0.325158, 0.341842, 0.35837, 0.37462, 0.390494, 0.406, 0.421147, 0.435943, 0.450397, 0.464515, 0.478307, 0.491779, 0.504939, 0.517794, 0.530351, 0.542618, 0.5546, 0.566305, 0.577738, 0.588907, 0.599817, 0.610474, 0.620885, 0.631054, 0.640988, 0.650691, 0.66017, 0.669429, 0.678474, 0.687309, 0.69594, 0.70437, 0.712606, 0.72065, 0.728508, 0.736185, 0.743683, 0.751007, 0.758162, 0.765152, 0.771979, 0.778648, 0.785163, 0.791527, 0.797743, 0.803815, 0.809747, 0.815541, 0.821201, 0.82673, 0.832131, 0.837407, 0.84256, 0.847594, 0.852512, 0.857315, 0.862008, 0.866591, 0.871069, 0.875443, 0.879715, 0.883889, 0.887965, 0.891948, 0.895838, 0.899638, 0.90335, 0.906976, 0.910518, 0.913977, 0.917357, 0.920659, 0.923884, 0.927034, 0.930111, 0.933117, 0.936054, 0.938922, 0.941724, 0.944461, 0.947135, 0.949746, 0.952297, 0.95479, 0.957224, 0.959602, 0.961925, 0.964194, 0.96641, 0.968575, 0.97069, 0.972756, 0.974775, 0.976746, 0.978672, 0.980553, 0.98239, 0.984185, 0.985939, 0.987652, 0.989325, 0.990959, 0.992555, 0.994115, 0.995638, 0.997126, 0.99858, 1.0] ("Init Data Out") w26] -> w24
            frame Disabled {
              # "T = 100"
            }
            frame Enabled {
              n9 = disable-structure shown="Enabled" {
                disable-tunnel: [sgl[] [0.0, 0.00863689, 0.0177355, 0.0273206, 0.0374182, 0.0480556, 0.059247, 0.0709632, 0.0831448, 0.095731, 0.108661, 0.121877, 0.135323, 0.148947, 0.162702, 0.176546, 0.190441, 0.204357, 0.218266, 0.232147, 0.245985, 0.259766, 0.273484, 0.287135, 0.300717, 0.314234, 0.32769, 0.341093, 0.354452, 0.367777, 0.381081, 0.394375, 0.407674, 0.420992, 0.434341, 0.447737, 0.461191, 0.474716, 0.488323, 0.502022, 0.515821, 0.529724, 0.543736, 0.557856, 0.572081, 0.586402, 0.600808, 0.615283, 0.629805, 0.644345, 0.658871, 0.673344, 0.687718, 0.701944, 0.715965, 0.72972, 0.743147, 0.756177, 0.768744, 0.780781, 0.792238, 0.803114, 0.813438, 0.823238, 0.83254, 0.841371, 0.849753, 0.85771, 0.865263, 0.872433, 0.879239, 0.885699, 0.891832, 0.897653, 0.903179, 0.908425, 0.913404, 0.918131, 0.922618, 0.926877, 0.93092, 0.934757, 0.9384, 0.941858, 0.945141, 0.948257, 0.951215, 0.954022, 0.956688, 0.959218, 0.961619, 0.963899, 0.966063, 0.968117, 0.970067, 0.971918, 0.973675, 0.975343, 0.976926, 0.978429, 0.979856, 0.98121, 0.982495, 0.983715, 0.984874, 0.985973, 0.987017, 0.988008, 0.988948, 0.989841, 0.990688, 0.991493, 0.992256, 0.992981, 0.993669, 0.994322, 0.994942, 0.995531, 0.99609, 0.99662, 0.997123, 0.997601, 0.998055, 0.998485, 0.998894, 0.999282, 0.99965, 1.0] ("Init Data Out") w28] -> w26
                frame Disabled {
                  # "T = 30"
                }
                frame Enabled {
                  n10 = disable-structure shown="Enabled" {
                    disable-tunnel: [sgl[] [0.0, 7.18341e-06, 1.77998e-05, 3.34898e-05, 5.66781e-05, 9.09483e-05, 0.000141596, 0.000216449, 0.000327074, 0.000490568, 0.000732196, 0.00108818, 0.00160286, 0.00232691, 0.00331916, 0.00464534, 0.00637594, 0.00858334, 0.0113384, 0.0147065, 0.018744, 0.0234947, 0.0289869, 0.0352312, 0.0422199, 0.0499271, 0.0583093, 0.0673079, 0.0768517, 0.0868599, 0.0972457, 0.107919, 0.118792, 0.129776, 0.140791, 0.151763, 0.162627, 0.173325, 0.18381, 0.194044, 0.203998, 0.21365, 0.222987, 0.232003, 0.240696, 0.24907, 0.257133, 0.264897, 0.272375, 0.279584, 0.286542, 0.293267, 0.299778, 0.306097, 0.312243, 0.318237, 0.324099, 0.32985, 0.33551, 0.341101, 0.346642, 0.352154, 0.357659, 0.363176, 0.368728, 0.374337, 0.380026, 0.385817, 0.391736, 0.397808, 0.40406, 0.41052, 0.417219, 0.424187, 0.431457, 0.439066, 0.447049, 0.455444, 0.464293, 0.473636, 0.483515, 0.493973, 0.505054, 0.516798, 0.529244, 0.54243, 0.556386, 0.571137, 0.586698, 0.603073, 0.620255, 0.63822, 0.656925, 0.676309, 0.696287, 0.716756, 0.737584, 0.758622, 0.779699, 0.800628, 0.821208, 0.841235, 0.860504, 0.878821, 0.896007, 0.911909, 0.926408, 0.939421, 0.950908, 0.960869, 0.969349, 0.976426, 0.982213, 0.986842, 0.990462, 0.993225, 0.995283, 0.996775, 0.997829, 0.998552, 0.999042, 0.999373, 0.999597, 0.999749, 0.999852, 0.999921, 0.999968, 1.0] ("Init Data Out") w30] -> w28
                    frame Disabled {
                      # "T = 30 alpha = 1"
                    }
                    frame Enabled {
                      n11 = disable-structure shown="Enabled" {
                        disable-tunnel: [sgl[] [0.0, 0.0224198, 0.0479575, 0.0767431, 0.108235, 0.14152, 0.175788, 0.210405, 0.244938, 0.279143, 0.31294, 0.34637, 0.379563, 0.412702, 0.445996, 0.479649, 0.513835, 0.548659, 0.584125, 0.620093, 0.656237, 0.692015, 0.726667, 0.759255, 0.788647, 0.814451, 0.837104, 0.856992, 0.874451, 0.889779, 0.903236, 0.915049, 0.925421, 0.934526, 0.94252, 0.949537, 0.955698, 0.961107, 0.965855, 0.970024, 0.973684, 0.976897, 0.979717, 0.982194, 0.984368, 0.986276, 0.987952, 0.989423, 0.990714, 0.991848, 0.992843, 0.993717, 0.994484, 0.995158, 0.995749, 0.996268, 0.996724, 0.997124, 0.997475, 0.997783, 0.998054, 0.998291, 0.9985, 0.998683, 0.998844, 0.998985, 0.999109, 0.999218, 0.999313, 0.999397, 0.999471, 0.999536, 0.999592, 0.999642, 0.999686, 0.999724, 0.999758, 0.999788, 0.999814, 0.999836, 0.999856, 0.999874, 0.999889, 0.999903, 0.999915, 0.999925, 0.999934, 0.999942, 0.99995, 0.999956, 0.999961, 0.999966, 0.99997, 0.999974, 0.999977, 0.99998, 0.999982, 0.999985, 0.999986, 0.999988, 0.99999, 0.999991, 0.999992, 0.999993, 0.999994, 0.999995, 0.999995, 0.999996, 0.999997, 0.999997, 0.999997, 0.999998, 0.999998, 0.999998, 0.999999, 0.999999, 0.999999, 0.999999, 0.999999, 0.999999, 1.0, 1.0, 1.0, 1.0, 1.0, 1.0, 1.0, 1.0] ("Init Data Out") sgl[] [0.0, 0.00121542, 0.00379376, 0.00667483, 0.00987316, 0.0134013, 0.0172697, 0.0214864, 0.0260568, 0.0309838, 0.0362677, 0.0419059, 0.0478934, 0.0542226, 0.0608838, 0.0678649, 0.0751518, 0.082729, 0.0905794, 0.0986844, 0.107025, 0.115581, 0.124333, 0.133259, 0.14234, 0.151554, 0.160883, 0.170308, 0.179809, 0.18937, 0.198974, 0.208606, 0.218251, 0.227896, 0.23753, 0.247141, 0.256719, 0.266257, 0.275747, 0.285183, 0.294559, 0.303872, 0.313117, 0.322293, 0.331399, 0.340432, 0.349393, 0.358283, 0.367102, 0.375854, 0.384538, 0.393159, 0.40172, 0.410223, 0.418672, 0.427073, 0.435428, 0.443742, 0.452021, 0.460268, 0.468489, 0.476689, 0.484874, 0.493047, 0.501216, 0.509384, 0.517558, 0.525742, 0.533942, 0.542163, 0.550411, 0.558689, 0.567004, 0.575359, 0.583759, 0.592209, 0.600712, 0.609272, 0.617893, 0.626578, 0.635329, 0.644148, 0.653038, 0.662, 0.671033, 0.680138, 0.689314, 0.698559, 0.707872, 0.717248, 0.726684, 0.736174, 0.745712, 0.755291, 0.764902, 0.774535, 0.78418, 0.793825, 0.803457, 0.813061, 0.822622, 0.832123, 0.841548, 0.850877, 0.860092, 0.869172, 0.878099, 0.88685, 0.895406, 0.903747, 0.911852, 0.919702, 0.927279, 0.934566, 0.941547, 0.948209, 0.954538, 0.960525, 0.966164, 0.971447, 0.976374, 0.980945, 0.985161, 0.98903, 0.992558, 0.995756, 0.998637, 1.0] ("Init Data Out")] -> w30
                        frame Disabled {
                          # "T = 30 alpha = 9"
                        }
                        frame Enabled {
                          # "T = 12 alpha =1"
                        }
                      }
                    }
                  }
                }
              }
            }
          }
        }
        frame 2 {
          # "Mpemba"
          # "Hot"
          n12 = disable-structure shown="Enabled" {
            disable-tunnel: [sgl[] [0.0, 0.00861236, 0.0172449, 0.0258978, 0.0345675, 0.043251, 0.0519446, 0.0606415, 0.0693372, 0.0780292, 0.0867166, 0.0953999, 0.10408, 0.11276, 0.121441, 0.130125, 0.138814, 0.14751, 0.156212, 0.164919, 0.173627, 0.182331, 0.191027, 0.199708, 0.208369, 0.21701, 0.22563, 0.23423, 0.24281, 0.25137, 0.25991, 0.26843, 0.27693, 0.28541, 0.29387, 0.302311, 0.310731, 0.319132, 0.327514, 0.335875, 0.344218, 0.35254, 0.360843, 0.369127, 0.377391, 0.385636, 0.393862, 0.402068, 0.410255, 0.418423, 0.426572, 0.434702, 0.442812, 0.450904, 0.458977, 0.467031, 0.475066, 0.483082, 0.49108, 0.499058, 0.507019, 0.51496, 0.522883, 0.530787, 0.538673, 0.54654, 0.554389, 0.56222, 0.570032, 0.577826, 0.585602, 0.593359, 0.601098, 0.60882, 0.616523, 0.624208, 0.631875, 0.639524, 0.647155, 0.654769, 0.662364, 0.669942, 0.677502, 0.685045, 0.692569, 0.700076, 0.707566, 0.715038, 0.722492, 0.729929, 0.737349, 0.744751, 0.752136, 0.759504, 0.766854, 0.774187, 0.781503, 0.788802, 0.796084, 0.803349, 0.810596, 0.817827, 0.825041, 0.832238, 0.839418, 0.846581, 0.853728, 0.860858, 0.867971, 0.875067, 0.882147, 0.88921, 0.896257, 0.903287, 0.910301, 0.917298, 0.924279, 0.931244, 0.938192, 0.945124, 0.95204, 0.95894, 0.965823, 0.972691, 0.979542, 0.986377, 0.993197, 1.0] ("Init Data Out") w35] -> w33
            frame Disabled {
              # "T = 1000"
            }
            frame Enabled {
              n13 = disable-structure shown="Enabled" {
                disable-tunnel: [sgl[] [0.0, 0.00908113, 0.0184019, 0.0279685, 0.0377876, 0.0478657, 0.058203, 0.0687801, 0.0795654, 0.0905285, 0.101641, 0.112875, 0.124206, 0.135613, 0.147074, 0.158572, 0.170092, 0.181619, 0.193144, 0.204658, 0.216154, 0.227626, 0.239071, 0.250489, 0.261878, 0.27324, 0.284576, 0.295889, 0.307184, 0.318465, 0.329736, 0.341004, 0.352273, 0.363551, 0.374842, 0.386152, 0.397487, 0.408852, 0.420252, 0.431689, 0.443169, 0.454692, 0.466259, 0.477871, 0.489526, 0.501221, 0.512951, 0.524708, 0.536484, 0.548268, 0.560046, 0.571802, 0.583519, 0.595174, 0.606745, 0.618207, 0.62953, 0.640684, 0.651639, 0.66236, 0.672819, 0.68301, 0.692938, 0.702611, 0.712036, 0.721218, 0.730165, 0.738881, 0.747373, 0.755647, 0.763708, 0.771562, 0.779215, 0.78667, 0.793934, 0.801011, 0.807906, 0.814624, 0.821169, 0.827546, 0.83376, 0.839813, 0.845711, 0.851457, 0.857055, 0.86251, 0.867824, 0.873002, 0.878047, 0.882961, 0.88775, 0.892416, 0.896961, 0.90139, 0.905705, 0.909909, 0.914005, 0.917995, 0.921883, 0.925672, 0.929362, 0.932958, 0.936462, 0.939875, 0.943201, 0.946441, 0.949598, 0.952673, 0.95567, 0.958589, 0.961434, 0.964205, 0.966906, 0.969536, 0.9721, 0.974597, 0.97703, 0.9794, 0.98171, 0.98396, 0.986153, 0.988289, 0.99037, 0.992397, 0.994373, 0.996298, 0.998173, 1.0] ("Init Data Out") w37] -> w35
                frame Disabled {
                  # "T = 60"
                }
                frame Enabled {
                  n14 = disable-structure shown="Enabled" {
                    disable-tunnel: [sgl[] [0.0, 0.00637855, 0.0128407, 0.0193875, 0.0260202, 0.0327398, 0.0395474, 0.0464443, 0.0534315, 0.0605103, 0.0676819, 0.0749469, 0.0823023, 0.0897424, 0.0972615, 0.104854, 0.112515, 0.120238, 0.128019, 0.135853, 0.143734, 0.151658, 0.159621, 0.167618, 0.175646, 0.183699, 0.191776, 0.199871, 0.207982, 0.216107, 0.224241, 0.232383, 0.24053, 0.248679, 0.256829, 0.264979, 0.273125, 0.281268, 0.289405, 0.297535, 0.305658, 0.313772, 0.321878, 0.329974, 0.33806, 0.346136, 0.354202, 0.362258, 0.370304, 0.37834, 0.386366, 0.394384, 0.402392, 0.410393, 0.418386, 0.426373, 0.434354, 0.44233, 0.450301, 0.458269, 0.466235, 0.474199, 0.482163, 0.490128, 0.498094, 0.506063, 0.514036, 0.522014, 0.529997, 0.537987, 0.545985, 0.553992, 0.562008, 0.570035, 0.578073, 0.586123, 0.594187, 0.602263, 0.610354, 0.61846, 0.626581, 0.634717, 0.642869, 0.651036, 0.65922, 0.667419, 0.675634, 0.683864, 0.692108, 0.700367, 0.708639, 0.716923, 0.725219, 0.733524, 0.741838, 0.750158, 0.758483, 0.766812, 0.77514, 0.783467, 0.791789, 0.800103, 0.808407, 0.816696, 0.824968, 0.833219, 0.841444, 0.849639, 0.8578, 0.865922, 0.874001, 0.882031, 0.890007, 0.897923, 0.905775, 0.913555, 0.921259, 0.928881, 0.936414, 0.943852, 0.951195, 0.958442, 0.965596, 0.972657, 0.979627, 0.986507, 0.993297, 1.0] ("Init Data Out") w39] -> w37
                    frame Disabled {
                      # "T = 60 alpha = 1"
                    }
                    frame Enabled {
                      n15 = disable-structure shown="Enabled" {
                        disable-tunnel: [sgl[] [0.0, 0.0217254, 0.0449123, 0.0695332, 0.0952912, 0.121775, 0.148649, 0.175659, 0.202636, 0.229485, 0.256173, 0.282716, 0.309165, 0.335592, 0.362081, 0.388712, 0.415553, 0.442644, 0.469983, 0.497515, 0.525114, 0.552573, 0.579595, 0.605797, 0.630672, 0.653979, 0.675818, 0.696279, 0.715452, 0.733415, 0.750247, 0.766017, 0.780794, 0.794639, 0.807611, 0.819766, 0.831155, 0.841826, 0.851824, 0.861192, 0.86997, 0.878194, 0.8859, 0.89312, 0.899885, 0.906224, 0.912163, 0.917728, 0.922942, 0.927828, 0.932405, 0.936694, 0.940713, 0.944478, 0.948007, 0.951312, 0.95441, 0.957312, 0.960031, 0.962579, 0.964966, 0.967203, 0.969298, 0.971262, 0.973102, 0.974826, 0.976441, 0.977954, 0.979373, 0.980701, 0.981946, 0.983113, 0.984206, 0.98523, 0.986189, 0.987088, 0.98793, 0.98872, 0.989459, 0.990152, 0.990801, 0.99141, 0.99198, 0.992514, 0.993014, 0.993483, 0.993922, 0.994334, 0.99472, 0.995081, 0.995419, 0.995737, 0.996034, 0.996312, 0.996573, 0.996818, 0.997047, 0.997262, 0.997463, 0.997651, 0.997828, 0.997993, 0.998148, 0.998293, 0.99843, 0.998557, 0.998677, 0.998789, 0.998893, 0.998992, 0.999084, 0.99917, 0.999251, 0.999327, 0.999398, 0.999464, 0.999526, 0.999585, 0.999639, 0.999691, 0.999739, 0.999784, 0.999826, 0.999865, 0.999902, 0.999937, 0.99997, 1.0] ("Init Data Out") sgl[] [0.0, 0.00121542, 0.00379376, 0.00667483, 0.00987316, 0.0134013, 0.0172697, 0.0214864, 0.0260568, 0.0309838, 0.0362677, 0.0419059, 0.0478934, 0.0542226, 0.0608838, 0.0678649, 0.0751518, 0.082729, 0.0905794, 0.0986844, 0.107025, 0.115581, 0.124333, 0.133259, 0.14234, 0.151554, 0.160883, 0.170308, 0.179809, 0.18937, 0.198974, 0.208606, 0.218251, 0.227896, 0.23753, 0.247141, 0.256719, 0.266257, 0.275747, 0.285183, 0.294559, 0.303872, 0.313117, 0.322293, 0.331399, 0.340432, 0.349393, 0.358283, 0.367102, 0.375854, 0.384538, 0.393159, 0.40172, 0.410223, 0.418672, 0.427073, 0.435428, 0.443742, 0.452021, 0.460268, 0.468489, 0.476689, 0.484874, 0.493047, 0.501216, 0.509384, 0.517558, 0.525742, 0.533942, 0.542163, 0.550411, 0.558689, 0.567004, 0.575359, 0.583759, 0.592209, 0.600712, 0.609272, 0.617893, 0.626578, 0.635329, 0.644148, 0.653038, 0.662, 0.671033, 0.680138, 0.689314, 0.698559, 0.707872, 0.717248, 0.726684, 0.736174, 0.745712, 0.755291, 0.764902, 0.774535, 0.78418, 0.793825, 0.803457, 0.813061, 0.822622, 0.832123, 0.841548, 0.850877, 0.860092, 0.869172, 0.878099, 0.88685, 0.895406, 0.903747, 0.911852, 0.919702, 0.927279, 0.934566, 0.941547, 0.948209, 0.954538, 0.960525, 0.966164, 0.971447, 0.976374, 0.980945, 0.985161, 0.98903, 0.992558, 0.995756, 0.998637, 1.0] ("Init Data Out")] -> w39
                        frame Disabled {
                          # "T = 60 alpha = 9"
                        }
                        frame Enabled {
                          # "T = 1000 alpha = 1"
                        }
                      }
                    }
                  }
                }
              }
            }
          }
        }
      }
    }
  }
  n16 = disable-structure shown="Enabled" {
    disable-tunnel: [w42 w45] -> w4
    frame Disabled {
      n17 = Random Number (0-1)() -> (number: 0 to 1=w42:dbl)
    }
    frame Enabled {
      # "1/32768"
      n18 = node-c288() -> (w44:T1)  [unwired: 1 in]
      n19 = timed-loop {
        timing: w44 -> [_]
        timing-out: [_] -> w43
        tunnel: [w51] -> w49
        stop <- TRUE stop-if-true
        n20 = call "White Noise Generator"() -> ("white noise out"=w51:i16)  [unwired: 15 in]
      }
      n21 = node-c288(w43) -> ()
      n22 = To Single Precision Float(number=w49) -> (single precision float=w47:sgl)
      n23 = Absolute Value(x=w47) -> (abs(x)=w46:sgl)
      n24 = Multiply(x=w46, y=sgl 3.051e-05) -> (x*y=w45:sgl)
    }
  }
  n25 = Array Size(array=w1) -> (size(s)=w3:i32)
  n26 = Decrement(x=w3) -> (x-1=w5:i32)
  n27 = while {
    tunnel: w1 -> [w93]
    tunnel: w4 -> [w74]
    shift-right: [w103] -> _
    shift-left: w5 -> [w94]
    shift-right: [w99] -> _
    shift-left: 0 -> [w95]
    shift-right: [w85] -> _
    shift-left: 0 -> [_]
    shift-right: [w96] -> _
    shift-left: w3 -> [w97]
    tunnel: [w93] -> _
    tunnel: w3 -> [w79]
    stop <- w101 stop-if-true
    w67 = sgl 305.0 ("y")
    w104 = -1  # floor-divide by 2
    # "x"
    # "x = (y-c)/m"
    # "c"
    # "m"
    # "y = mx+c"
    # "m"
    n28 = Add(x=w94, y=w95) -> (x+y=w100:i32)
    n29 = Greater?(x=w95, y=w94) -> (0:w102:bool)
    n30 = Greater?(x=w74, y=sgl 0.99999) -> (0:w64:bool)
    n31 = Logical Shift(y=w104, x=w100) -> (x << y=w91:i32)
    n32 = Index Array(array=w93, index=w91) -> (element=w63:sgl)
    n33 = Index Array(array=w93, index=w91) -> (element=w59:sgl)
    n34 = Multiply(x="RN", y=w59) -> (x*y=w57:sgl)
    n35 = Multiply(x=w63, y="RN") -> (x*y=w62:sgl)
    n36 = Less?(x=w62, y=w74) -> (x < y?=w98:bool)
    n37 = Equal?(x=w74, y=w62) -> (x = y?=w92:bool)
    n38 = Or(x=w92, y=w102) -> (x .or. y?=w101:bool)
    n39 = case shown="True" w98 {
      tunnel: w91 -> [w126 w129]
      tunnel: [w125 w127] -> w103
      tunnel: w95 -> [w124 _]
      tunnel: [w124 w128] -> w99
      tunnel: w94 -> [_ w127]
      frame False {
        n40 = Decrement(x=w126) -> (x-1=w125:i32)
      }
      frame True {
        n41 = Increment(x=w129) -> (x+1=w128:i32)
      }
    }
    n42 = case shown="True" w98 {
      tunnel: w91 -> [w120 w123]
      tunnel: [w119 w122] -> w85
      tunnel: w97 -> [w119 w121]
      tunnel: [w120 w121] -> w96
      frame False {
      }
      frame True {
        n43 = Increment(x=w123) -> (x+1=w122:i32)
      }
    }
    n44 = To Single Precision Float(number=w79) -> (single precision float=w78:sgl)
    n45 = disable-structure shown="Enabled" {
      disable-tunnel: [w105 w108] -> w69
      frame Disabled {
        n46 = Random Number (0-1)() -> (number: 0 to 1=w105:dbl)
      }
      frame Enabled {
        n47 = node-c288() -> (w107:T1)  [unwired: 1 in]
        n48 = timed-loop {
          timing: w107 -> [_]
          timing-out: [_] -> w106
          tunnel: [w114] -> w112
          stop <- TRUE stop-if-true
          n49 = call "White Noise Generator2"() -> ("white noise out"=w114:i16)  [unwired: 15 in]
        }
        n50 = node-c288(w106) -> ()
        n51 = To Single Precision Float(number=w112) -> (single precision float=w110:sgl)
        n52 = Absolute Value(x=w110) -> (abs(x)=w109:sgl)
        n53 = Multiply(x=w109, y=sgl 3.051e-05) -> (x*y=w108:sgl)
      }
    }
    n54 = Index Array(array=w93, index=w85) -> (element=w61:sgl)
    n55 = Multiply(x=w61, y="RN") -> (x*y=w60:sgl)
    n56 = Subtract(x=w60, y=w57) -> (x-y=w87:sgl)
    n57 = Multiply(x=w87, y=w85) -> (x*y=w90:sgl)
    n58 = Subtract(x=w60, y=w90) -> (x-y=w89:sgl)
    n59 = Subtract(x=w74, y=w89) -> (x-y=w88:sgl)
    n60 = Subtract(x=sgl 1024.0, y=w67) -> (x-y=w70:sgl)
    n61 = Divide(x=w88, y=w87) -> (x/y=w86:sgl)
    n62 = Multiply(x=w70, y=w69) -> (x*y=w68:sgl)
    n63 = Multiply(x=sgl 12.0, y="X0") -> (x*y=w82:sgl)
    n64 = Multiply(x="X0", y=sgl -2.0) -> (x*y=w76:sgl)
    n65 = Add(x=w68, y=w67) -> (x+y=w65:sgl)
    n66 = Subtract(x=w82, y=w76) -> (x-y=w81:sgl)
    n67 = Select(t=w91, s=w92, f=w86) -> (s? t:f=w72:sgl)
    n68 = Divide(x=w81, y=w78) -> (x/y=w80:sgl)
    n69 = Select(t=w65, s=w64, f=w72) -> (s? t:f=w66:sgl)
    n70 = Multiply(x=w66, y=w80) -> (x*y=w77:sgl)
    n71 = Add(x=w77, y=w76) -> (x+y=→"Xpot":sgl)
  }
